vi "SW_Draw_mouse_br.vi"(0 "Input picture (background)":picture, 1 "Size of the image":T1={"Numeric Control"=480.0, "Numeric Control"=480.0}, 5 "Pixels per mm":dbl=2.0, 7 "Mouse coord cartesian X, mm":dbl, 9 "Mouse coord cartesian Y, mm":dbl, 11 "Mouse angle of rotation, deg":dbl=200.0, 12 "Show mouse lineout":bool, 13 "Trace length, samples":u16=20 max=1000 step=1) -> (4 "Output picture (with mouse overlay)":picture, 6 "Mouse abs. coordinates, pix":T1={"Numeric Control"=240.0, "Numeric Control"=240.0})   [LabVIEW 2018, in "Tracker.lvlib"]
uses:
  Tracker.lvlib
  <vilib>/Utility/miscctls.llb/LVBoundsTypeDef.ctl
panel:
  in  "Choose trace style":bool=TRUE
  out "Time per draw":dbl
  out "Colors array output":u32[](array[colorbox])
  in  "Colors array input":u32[](array[colorbox])=[255, 65535, 6618880, 16776960, 16744448, 16711680]
  in  "Rainbow colors":bool
  in  "Trace color 2":u32(colorbox)
  in  "Trace color":u32(colorbox)=16757314
  in  "Mouse lineout color":u32(colorbox)=16775210
  in  "Iris size factor":dbl=0.05000000000000001 min=0.01 max=0.22 step=0.005 format="%#_13g"
  in  "Eye size factor":dbl=0.07000000000000002 min=0.02 max=0.24 step=0.01 format="%#_13g"
  in  "Mouse color":u32(colorbox)=5460819
  in  "Mouse length, mm":dbl=40.0
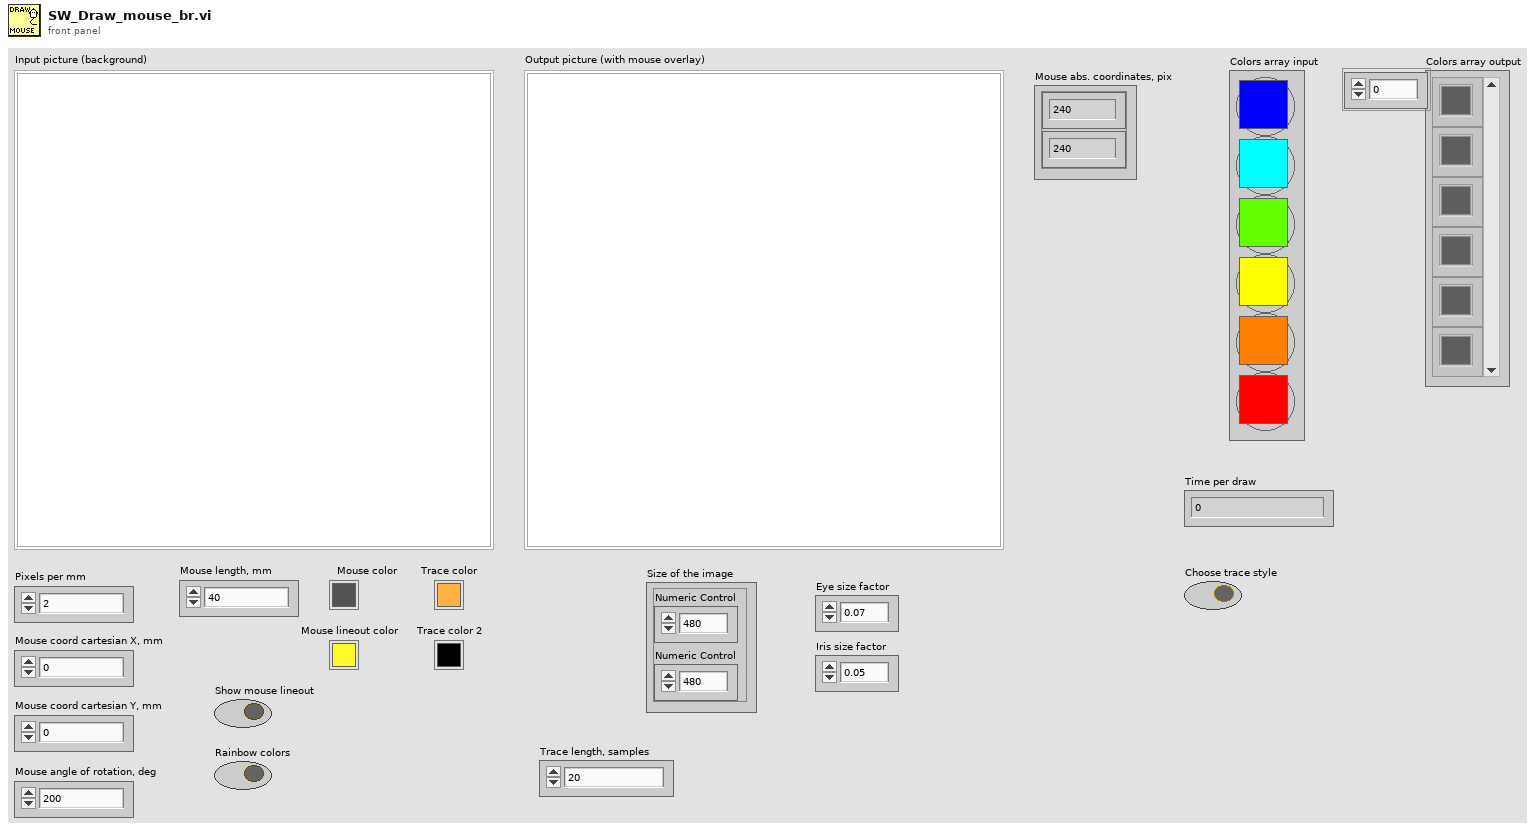
[diagram p1: front panel]
types:
  T1 = cluster{"Numeric Control":dbl, "Numeric Control":dbl}
  T2 = cluster{"Width":u16, "Style":enum32{"Solid", "Dash", "Dot", "DashDot", "DashDotDot"}}
  T3 = typedef "LVBoundsTypeDef.ctl" = cluster{"Width":u32, "Height":u32}
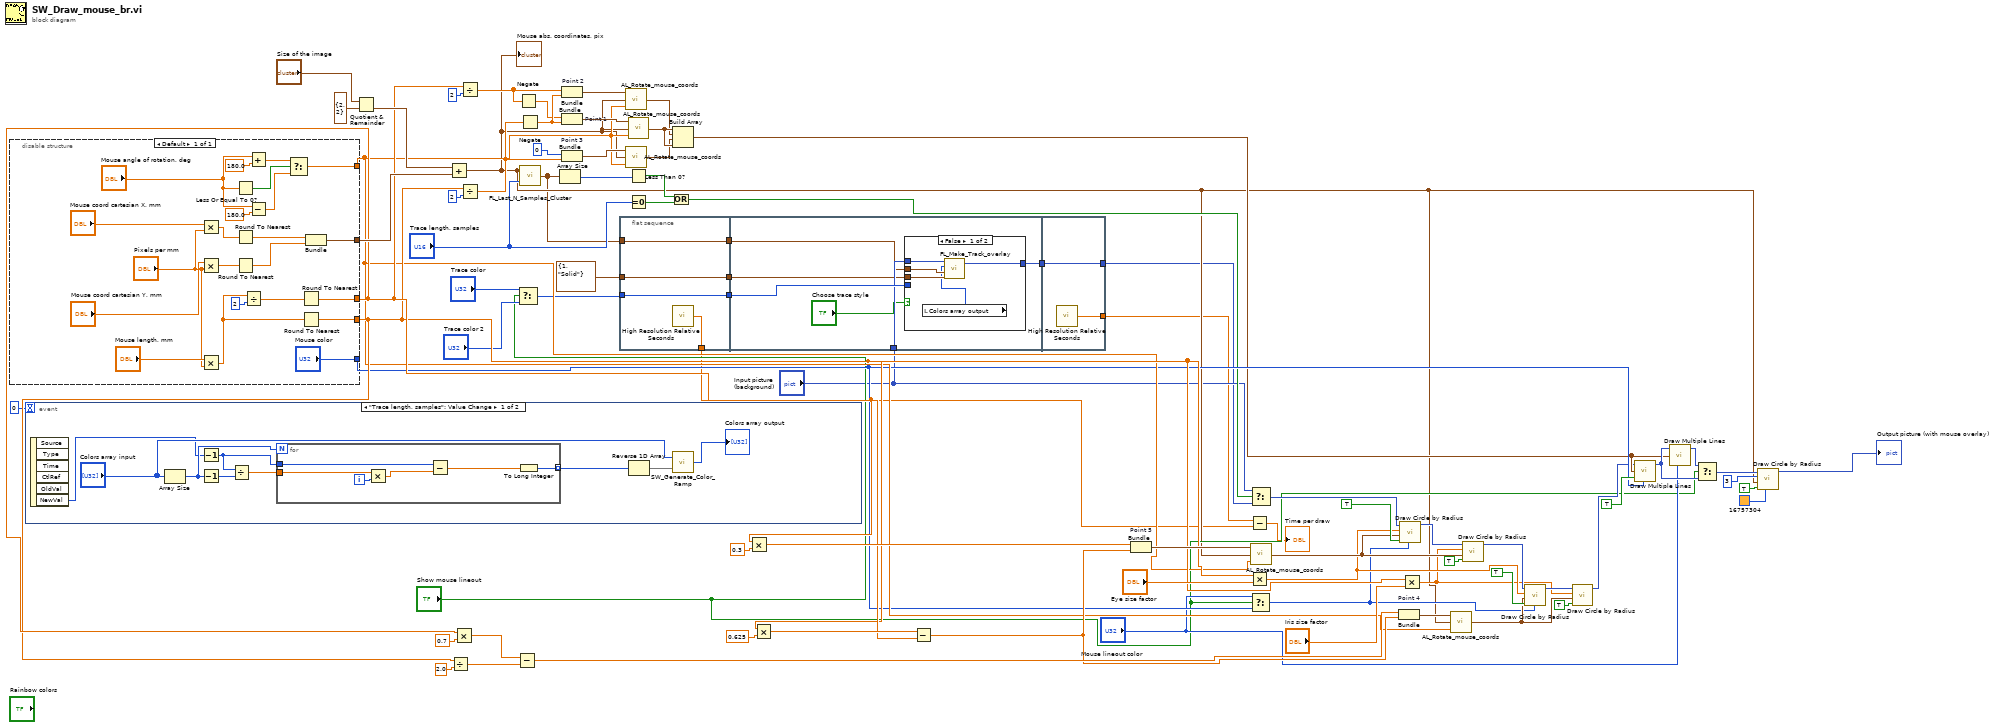
[diagram p0: block diagram]
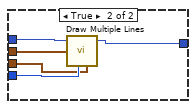
[diagram p2: hidden frame]
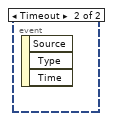
[diagram p3: hidden frame]
diagram:
  n1 = disable-structure shown="Default" {
    disable-tunnel: ["Mouse color"] -> w33
    disable-tunnel: [w97] -> w42
    disable-tunnel: [w99] -> w40
    disable-tunnel: [w82] -> w38
    disable-tunnel: [w89] -> w55
    frame Enabled {
      n2 = Multiply(x="Mouse coord cartesian X, mm", y="Pixels per mm") -> (x*y=w95:dbl)
      n3 = Multiply(x="Mouse coord cartesian Y, mm", y="Pixels per mm") -> (x*y=w94:dbl)
      n4 = Multiply(x="Mouse length, mm", y="Pixels per mm") -> (x*y=w100:dbl)
      n5 = Less Or Equal To 0?(x="Mouse angle of rotation, deg") -> (x <= 0?=w88:bool)
      n6 = Round To Nearest(number=w95) -> (nearest integer value=w91:dbl)
      n7 = Round To Nearest(number=w94) -> (nearest integer value=w90:dbl)
      n8 = Divide(x=w100, y=2) -> (x/y=w98:dbl)
      n9 = Add(x="Mouse angle of rotation, deg", y=sgl 180.0) -> (x+y=w85:dbl)
      n10 = Subtract(x="Mouse angle of rotation, deg", y=sgl 180.0) -> (x-y=w87:dbl)
      n11 = Select(t=w85, s=w88, f=w87) -> (s? t:f=w82:dbl)
      n12 = Round To Nearest(number=w98) -> (nearest integer value=w97:dbl)
      n13 = Round To Nearest(number=w100) -> (nearest integer value=w99:dbl)
      n14 = Bundle(w91, w90) -> (w89:cluster{dbl, dbl})  [unwired: 1 in]
    }
  }
  n15 = event shown="[0] \"Trace length, samples\": Value Change" {
    selector: _ -> [_ _]
    dyn-events: _ -> [_ _]
    timeout: 0 -> [_ _]
    event "Trace length, samples": Value Change {
      n16 = event-data() -> ("NewVal"=w105:u16)  [unwired: 1 in, 5 out]
      n17 = Array Size(array="Colors array input") -> (size(s)=w107:i32)
      n18 = Decrement(x=w105) -> (x-1=w108:u16)
      n19 = Decrement(x=w107) -> (x-1=w111:i32)
      n20 = Divide(x=w108, y=w111) -> (x/y=w112:dbl)
      n21 = for {
        N: w107 -> [_]
        tunnel: [w113] -> w110 mode=indexing
        tunnel: w108 -> [w118]
        tunnel: w112 -> [w116]
        i -> [w114]
        n22 = Multiply(x=w116, y=w114) -> (x*y=w117:dbl)
        n23 = Subtract(x=w118, y=w117) -> (x-y=w115:dbl)
        n24 = To Long Integer(number=w115) -> (32bit integer=w113:i32)
      }
      n25 = Reverse 1D Array(array=w110) -> (reversed array=w109:i32[])
      n26 = call "SW_Generate_Color_Ramp.vi"("Colors rel. pos."=w109, "Colors array"="Colors array input") -> ("Colors array"=→"Colors array output":u32[])
    }
    event Timeout {
      n27 = event-data() -> ()  [unwired: 1 in, 3 out]
    }
  }
  n28 = Quotient & Remainder(x="Size of the image", y=T3 {"Width"=2, "Height"=2}) -> (floor(x/y)=w54:cluster{dbl, dbl})  [unwired: 1 out]
  n29 = Add(x=w54, y=w55) -> (x+y=w16:cluster{dbl, dbl})
  "Mouse abs. coordinates, pix" <- w16
  n30 = Divide(x=w40, y=2.0) -> (x/y=w48:dbl)
  n31 = Multiply(x=w42, y=0.7) -> (x*y=w52:dbl)
  n32 = Divide(x=w42, y=u16 2) -> (x/y=w37:dbl)
  n33 = Divide(x=w40, y=u16 2) -> (x/y=w70:dbl)
  n34 = Subtract(x=w52, y=w48) -> (x-y=w51:dbl)
  n35 = Select(t="Trace color", s="Show mouse lineout", f="Trace color 2") -> (s? t:f=w22:u32)
  n36 = Negate(x=w37) -> (-x=w36:dbl)
  n37 = Negate(x=w70) -> (-x=w39:dbl)
  n38 = call "FL_Last_N_Samples_Cluster.vi"("BufferLengthSamples"="Trace length, samples", "Input cluster"=w16) -> ("Output 1D array of clusters"=w10:cluster{"X":dbl, "Y":dbl}[])
  n39 = Array Size(array=w10) -> (size(s)=w28:i32)
  n40 = Bundle "Point 2"(w37, w39) -> (w65:cluster{dbl, dbl})  [unwired: 1 in]
  n41 = Bundle "Point 1"(w36, w39) -> (w66:cluster{dbl, dbl})  [unwired: 1 in]
  n42 = Bundle "Point 3"(0, w70) -> (w64:cluster{i32, dbl})  [unwired: 1 in]
  n43 = flat-sequence {
    tunnel: w10 -> [w120]
    tunnel: T2 {"Width"=1, "Style"=enum."Solid"} ("pen") -> [w121]
    tunnel: w22 -> [w122]
    tunnel: [w122] -> w7
    tunnel: [w121] -> w6
    tunnel: [w120] -> w5
    tunnel: [w119] -> w3
    tunnel: "Input picture (background)" -> [w127]
    tunnel: [w126] -> w8
    tunnel: w7 -> [w128]
    tunnel: w6 -> [w125]
    tunnel: w5 -> [w124]
    tunnel: [w140] -> w12
    tunnel: w8 -> [w140]
    tunnel: [w139] -> w4
    frame #0 {
      n44 = call <vilib>:"High Resolution Relative Seconds.vi"() -> ("relative seconds"=w119:dbl)
    }
    frame #1 {
      n45 = case shown="False" "Choose trace style" {
        tunnel: w128 -> [_ w138]
        tunnel: w127 -> [w133 w137]
        tunnel: [w132 w136] -> w126
        tunnel: w125 -> [w131 w135]
        tunnel: w124 -> [w130 w134]
        frame False {
          n46 = local read "Colors array output"() -> (w129:u32[])
          n47 = call "FL_Make_Track_overlay.vi"("Pen properties"=w131, "Full track array"=w130, "Colors array input"=w129, "Picture in"=w133) -> ("Picture out"=w132:picture)  [unwired: 3 in]
        }
        frame True {
          n48 = call <vilib>:"Draw Multiple Lines.vi"("picture"=w137, "line endpoints"=w134, "color(black)"=w138, "pen"=w135) -> ("new picture"=w136:picture)  [unwired: 5 in]
        }
      }
    }
    frame #2 {
      n49 = call <vilib>:"High Resolution Relative Seconds.vi"() -> ("relative seconds"=w139:dbl)
    }
  }
  n50 = call "AL_Rotate_mouse_coords.vi"("Mouse angle of rotation, deg"=w38, "Offset"=w16, "Coordinates to rotate"=w65) -> ("Rotated coordinates"=w58:cluster{"X":dbl, "Y":dbl})
  n51 = call "AL_Rotate_mouse_coords.vi"("Mouse angle of rotation, deg"=w38, "Offset"=w16, "Coordinates to rotate"=w64) -> ("Rotated coordinates"=w57:cluster{"X":dbl, "Y":dbl})
  n52 = call "AL_Rotate_mouse_coords.vi"("Mouse angle of rotation, deg"=w38, "Offset"=w16, "Coordinates to rotate"=w66) -> ("Rotated coordinates"=w59:cluster{"X":dbl, "Y":dbl})
  n53 = Less Than 0?(x=w28) -> (x < 0?=w26:bool)
  n54 = Equal To 0?(x="Trace length, samples") -> (x = 0?=w25:bool)
  n55 = Or(x=w26, y=w25) -> (x .or. y?=w24:bool)
  n56 = Build Array(w59, w58, w57, w59) -> (w29:cluster{"X":dbl, "Y":dbl}[])
  n57 = Multiply(x=w42, y=0.3) -> (x*y=w46:dbl)
  n58 = Multiply(x=w40, y=0.625) -> (x*y=w49:dbl)
  n59 = Subtract(x=w49, y=w42) -> (x-y=w50:dbl)
  n60 = Bundle "Point 5"(w46, w50) -> (w62:cluster{dbl, dbl})  [unwired: 1 in]
  n61 = Subtract(x=w4, y=w3) -> (x-y=→"Time per draw":dbl)
  n62 = Multiply(x=w40, y="Eye size factor") -> (x*y=w44:dbl)
  n63 = Select(t="Mouse lineout color", s="Show mouse lineout", f=w33) -> (s? t:f=w31:u32)
  n64 = Select(t="Input picture (background)", s=w24, f=w12) -> (s? t:f=w19:picture)
  n65 = call "AL_Rotate_mouse_coords.vi"("Mouse angle of rotation, deg"=w38, "Offset"=w16, "Coordinates to rotate"=w62) -> ("Rotated coordinates"=w61:cluster{"X":dbl, "Y":dbl})
  n66 = Bundle "Point 4"(w51, w50) -> (w63:cluster{dbl, dbl})  [unwired: 1 in]
  n67 = call <vilib>:"Draw Circle by Radius.vi"("color(black)"=w31, "fill?(F)"=TRUE, "pixel center"=w61, "radius"=w44, "picture"=w19) -> ("new picture"=w77:picture)  [unwired: 6 in]
  n68 = Multiply(x=w40, y="Iris size factor") -> (x*y=w41:dbl)
  n69 = call "AL_Rotate_mouse_coords.vi"("Mouse angle of rotation, deg"=w38, "Offset"=w16, "Coordinates to rotate"=w63) -> ("Rotated coordinates"=w60:cluster{"X":dbl, "Y":dbl})
  n70 = call <vilib>:"Draw Circle by Radius.vi"("fill?(F)"=TRUE, "pixel center"=w61, "radius"=w41, "picture"=w77) -> ("new picture"=w76:picture)  [unwired: 7 in]
  n71 = call <vilib>:"Draw Circle by Radius.vi"("color(black)"=w31, "fill?(F)"=TRUE, "pixel center"=w60, "radius"=w44, "picture"=w76) -> ("new picture"=w74:picture)  [unwired: 6 in]
  n72 = call <vilib>:"Draw Circle by Radius.vi"("fill?(F)"=TRUE, "pixel center"=w60, "radius"=w41, "picture"=w74) -> ("new picture"=w20:picture)  [unwired: 7 in]
  n73 = call <vilib>:"Draw Multiple Lines.vi"("picture"=w20, "line endpoints"=w29, "fill?(F)"=TRUE, "color(black)"=w33) -> ("new picture"=w34:picture)  [unwired: 5 in]
  n74 = call <vilib>:"Draw Multiple Lines.vi"("picture"=w34, "line endpoints"=w29, "color(black)"="Mouse lineout color") -> ("new picture"=w30:picture)  [unwired: 6 in]
  n75 = Select(t=w30, s="Show mouse lineout", f=w34) -> (s? t:f=w35:picture)
  n76 = call <vilib>:"Draw Circle by Radius.vi"("color(black)"=u32 16757304, "fill?(F)"=TRUE, "pixel center"=w16, "radius"=i16 3, "picture"=w35) -> ("new picture"=→"Output picture (with mouse overlay)":picture)  [unwired: 6 in]
